vi "Set_Compliance_Slope_R2.vi"(8 "Compliance Slope":u8=128, 9 "DIO Ref Out":T1, 10 "VISA resource name":refnum<visa-resource-name>="ASRL1::INSTR", 11 "Servo ID":string="\u0001") -> (2 "Valid Checksum":bool=TRUE, 3 "Error":u64)   [LabVIEW 2015]
uses:
  <vilib>/myRIO/Instrument Drivers/Onboard IO/DIO/typedefs/DIO Reference.ctl
  <vilib>/myRIO/Common/Instrument Driver Framework/Utilities/typedefs/myRIO Generic Hardware Reference.ctl
  <vilib>/myRIO/Common/Instrument Driver Framework/Utilities/typedefs/Hardware Version Enum.ctl
  <vilib>/myRIO/Common/Instrument Driver Framework/Utilities/typedefs/myRIO v1.0 Reference.ctl
  <vilib>/myRIO/Common/Instrument Driver Framework/Utilities/typedefs/Generic FPGA Reference.ctl
  <vilib>/myRIO/Common/Instrument Driver Framework/myRIO v1.0/DIO/typedefs/DIO Channels List.ctl
  <vilib>/myRIO/Common/Instrument Driver Framework/myRIO v1.0/DIO/typedefs/DIO Channels Enum.ctl
  <vilib>/Utility/error.llb/Error Cluster From Error Code.vi
  <vilib>/myRIO/Common/Instrument Driver Framework/myRIO v1.0/DIO/vis/myRIO v1.0 Write DIO.vi
  <vilib>/myRIO/Instrument Drivers/Onboard IO/DIO/DIO.lvlib
panel:
  out "Valid Checksum 2":bool=TRUE
  out "Error 2":u64
  out "Received String 2":string
  out "Received String Array 2":string[](array[string])
  out "Received\nArray 2":u8[](array[numeric])
  out "Received\nCksm 2":u8
  out "Calc Cksm 2":u8
  in  "Return\nDelay (us) 2":i32=1000
  in  "RECEIVE (F) 2":bool[](array[boolean])=[FALSE]
  out "Tx Packet 2":string
  out "Checksum 2":string
  in  "Transmit \nDelay (us) 2":i32=850
  out "CS 2":string
  in  "TRANSMIT (T) 2":bool[](array[boolean])=[TRUE]
  out "CS":string
  out "Checksum":string
  out "Tx Packet":string
  out "Calc Cksm":u8
  out "Received\nCksm":u8
  out "Received\nArray":u8[](array[numeric])
  in  "Transmit \nDelay (us)":i32=850
  in  "Return\nDelay (us)":i32=1000
  in  "RECEIVE (F)":bool[](array[boolean])=[FALSE]
  in  "TRANSMIT (T)":bool[](array[boolean])=[TRUE]
  out "Received String Array":string[](array[string])
  out "Received String":string
  # "SEND VALUES"
  # "RECEIVED VALUES"
  # "OUTPUT VALUES"
  # "INPUT"
  # "Config Parameters"
  # "Tx/Rx Delays"
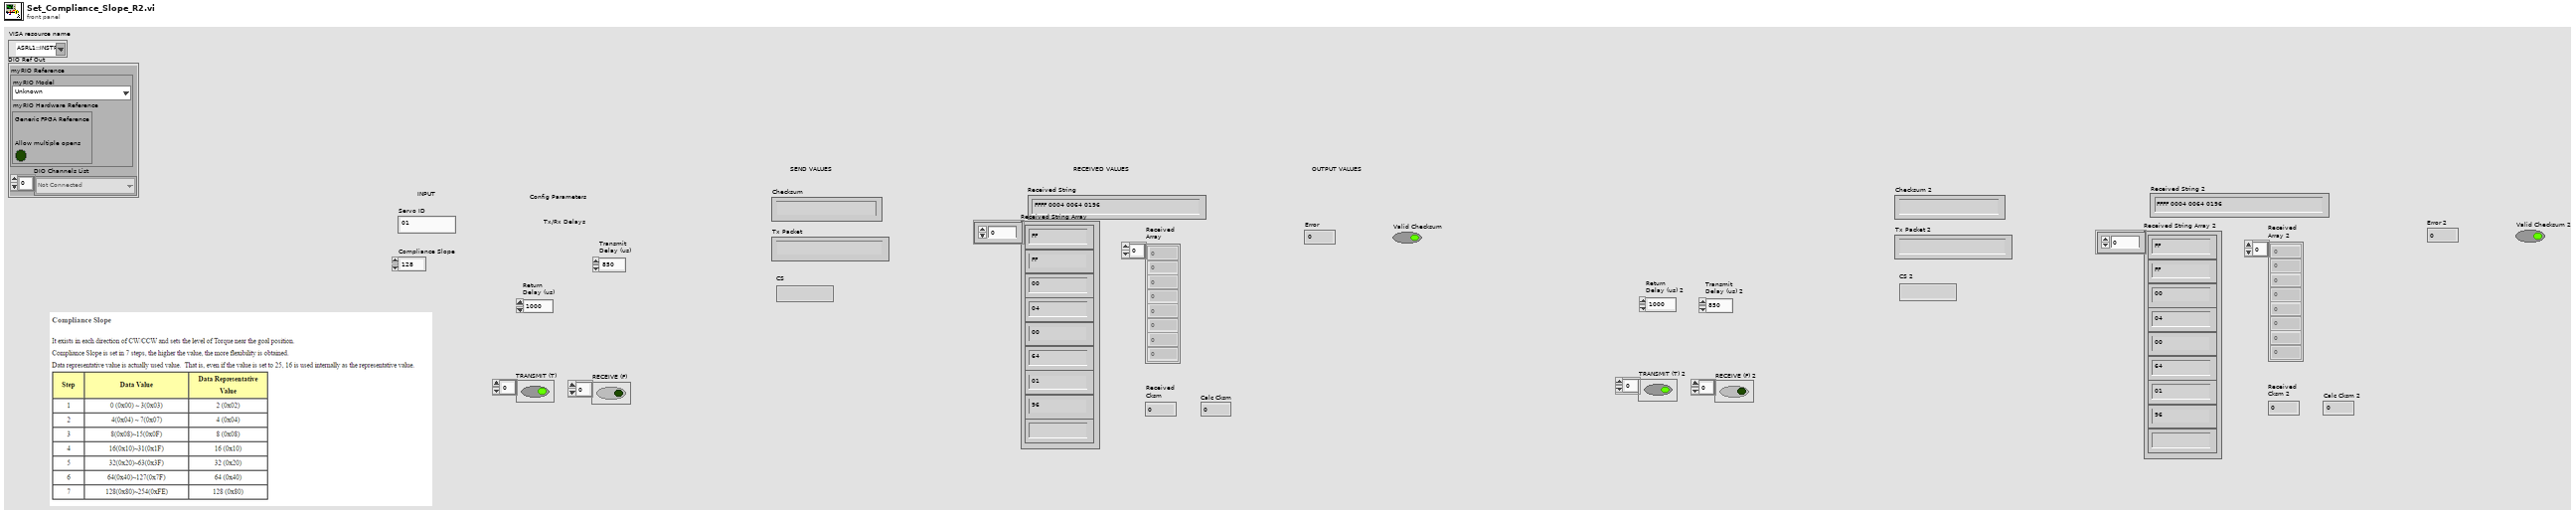
[diagram p1: front panel]
types:
  T1 = typedef "DIO.lvlib/DIO Reference.ctl" = cluster{"myRIO Reference":T2, "DIO Channels List":T6}
  T2 = typedef "myRIO Generic Hardware Reference.ctl" = cluster{"myRIO Model":T3, "myRIO Hardware Reference":T4}
  T3 = typedef "Hardware Version Enum.ctl" = enum16{"Unknown", "myRIO-1900", "myRIO-1950", "roboRIO"}
  T4 = typedef "myRIO v1.0 Reference.ctl" = cluster{"Generic FPGA Reference":T5, "Allow multiple opens":bool}
  T5 = typedef "Generic FPGA Reference.ctl" = refnum<k20>
  T6 = typedef "DIO Channels List.ctl" = T7[]
  T7 = typedef "DIO Channels Enum.ctl" = enum16{"Not Connected", "C/DIO0", "C/DIO1", "C/DIO2", "C/DIO3", "C/DIO4", "C/DIO5", "C/DIO6", "C/DIO7", "A/DIO0", "A/DIO1", "A/DIO2", "A/DIO3", "A/DIO4", "A/DIO5", "A/DIO6", "A/DIO7", "A/DIO8", "A/DIO9", "A/DIO10", "A/DIO11", "A/DIO12", "A/DIO13", "A/DIO14", "A/DIO15", "B/DIO0", "B/DIO1", "B/DIO2", "B/DIO3", "B/DIO4", "B/DIO5", "B/DIO6", "B/DIO7", "B/DIO8", "B/DIO9", "B/DIO10", "B/DIO11", "B/DIO12", "B/DIO13", "B/DIO14", "B/DIO15", "LED0", "LED1", "LED2", "LED3", "Button0", "DIO/DIO0", "DIO/DIO1", "DIO/DIO2", "DIO/DIO3", "DIO/DIO4", "DIO/DIO5", "DIO/DIO6", "DIO/DIO7", "DIO/DIO8", "DIO/DIO9", "SPI/CS0", "SPI/CS1", "SPI/CS2", "SPI/CS3", "LED RADIO (Green)", "LED RADIO (Red)", "LED COMM (Green)", "LED COMM (Red)", "LED MODE (Green)", "LED MODE (Red)"}
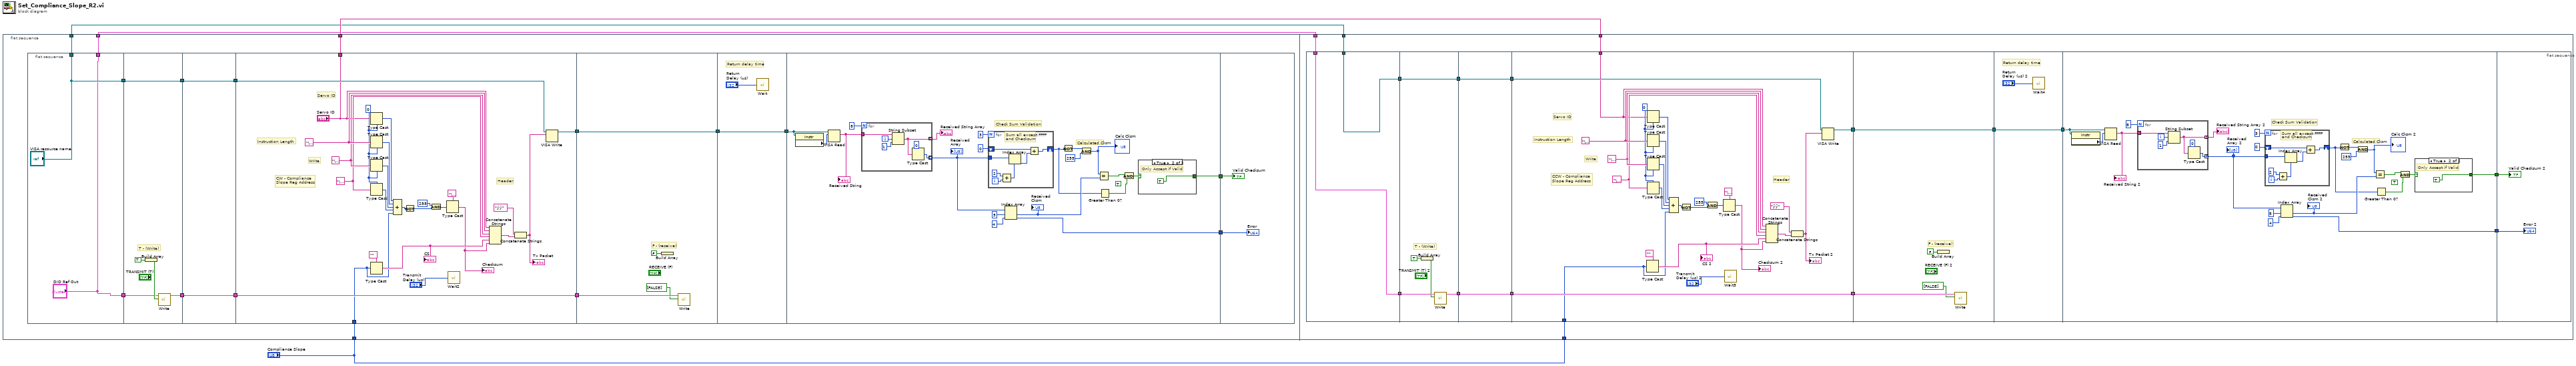
[diagram p0: block diagram]
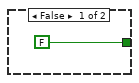
[diagram p2: hidden frame]
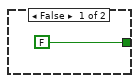
[diagram p3: hidden frame]
diagram:
  n1 = flat-sequence {
    tunnel: "Compliance Slope" -> [w8]
    tunnel: [w7] -> w3
    tunnel: [w5] -> w2
    tunnel: [w6] -> w1
    tunnel: "Compliance Slope" -> [w101]
    tunnel: w3 -> [w100]
    tunnel: w2 -> [w99]
    tunnel: w1 -> [w98]
    frame #0 {
      n2 = flat-sequence {
        tunnel: ["VISA resource name"] -> w20
        tunnel: ["DIO Ref Out"] -> w19
        tunnel: ["DIO Ref Out"] -> w6
        tunnel: ["VISA resource name"] -> w5
        tunnel: [w27] -> w18
        tunnel: [w25] -> w17
        tunnel: w20 -> [w25]
        tunnel: w19 -> [w23]
        tunnel: [w29] -> w16
        tunnel: w18 -> [w29]
        tunnel: [w28] -> w15
        tunnel: w17 -> [w28]
        tunnel: [w54] -> w13
        tunnel: w16 -> [w54]
        tunnel: w15 -> [w53]
        tunnel: [w52] -> w14
        tunnel: w8 -> [w31]
        tunnel: ["Servo ID"] -> w7
        tunnel: [w56] -> w12
        tunnel: w14 -> [w56]
        tunnel: w13 -> [w58]
        tunnel: w12 -> [w59]
        tunnel: [w59] -> w11
        tunnel: w11 -> [w78]
        tunnel: [w63] -> w10
        tunnel: [w61] -> w9
        tunnel: w10 -> [w97]
        tunnel: w9 -> [w96]
        frame #0 {
        }
        frame #1 {
          # "T - (Write)"
          n3 = Build Array(TRUE) -> (w24:bool[])
          n4 = call <vilib>:"Write.vi"("Values"=w24, "DIO Ref In"=w23) -> ("DIO Ref Out"=w27:T1)  [unwired: 7 in, 1 out]
        }
        frame #2 {
        }
        frame #3 {
          w39 = u8 0
          w34 = "\u001c"
          w43 = "\u0003"
          w44 = "\u0004"
          # "CW - Compliance\nSlope Reg Address"
          # "Write"
          # "Instruction Length"
          # "Servo ID"
          # "Header"
          n5 = Type Cast(type="", x=w31) -> (*(type *) &x=w33:string)
          "CS" <- w33
          n6 = Type Cast(type=w39, x="Servo ID") -> (*(type *) &x=w45:u8)
          n7 = Type Cast(type=w39, x=w44) -> (*(type *) &x=w46:u8)
          n8 = Type Cast(type=w39, x=w43) -> (*(type *) &x=w38:u8)
          n9 = Type Cast(type=w39, x=w34) -> (*(type *) &x=w47:u8)
          n10 = Compound Arithmetic op=ADD(w45, w46, w38, w47, w31) -> (w48:u8)
          n11 = Not(x=w48) -> (.not. x?=w50:u8)
          n12 = And(x=u8 255, y=w50) -> (x .and. y?=w51:u8)
          n13 = Type Cast(type="\u0000", x=w51) -> (*(type *) &x=w32:string)
          "Checksum" <- w32
          n14 = call "Wait2"("Count(uSec)"="Transmit \nDelay (us)") -> ()  [unwired: 1 out]
          n15 = Concatenate Strings("Servo ID", w44, w43, w34, w33, w32) -> (w41:string)
          n16 = Concatenate Strings("ÿÿ", w41) -> (w37:string)
          "Tx Packet" <- w37
          n17 = VISA Write(VISA resource name=w53, write buffer=w37) -> (VISA resource name out=w52:refnum<visa-resource-name>)  [unwired: 1 in, 2 out]
        }
        frame #4 {
          # "F - (receive)"
          n18 = Build Array(FALSE) -> ()  [unwired: 1 out]
          n19 = call <vilib>:"Write.vi"("Values"=bool[] [FALSE], "DIO Ref In"=w58) -> ()  [unwired: 7 in, 2 out]
        }
        frame #5 {
          # "Return delay time"
          n20 = call "Wait"("Count(uSec)"="Return\nDelay (us)") -> ()  [unwired: 1 out]
        }
        frame #6 {
          (unwired) TRUE
          # "Calculated Cksm"
          # "Check Sum Validation"
          n21 = property class="Instr"(reference=w78) -> ("Serial Settings:Number of Bytes at Serial Port"=w77:u32)  [unwired: 1 in, 2 out]
          n22 = VISA Read(VISA resource name=w78, byte count=w77) -> (read buffer=w79:string)  [unwired: 1 in, 3 out]
          "Received String" <- w79
          n23 = for {
            N: 8 -> [_]
            tunnel: w79 -> [w95]
            tunnel: [w91] -> w76 mode=indexing
            tunnel: [w90] -> w74 mode=indexing
            i -> [w94]
            n24 = String Subset(string=w95, offset (0)=w94, length (rest)=1) -> (substring=w91:string)
            n25 = Type Cast(type=u8 0, x=w91) -> (*(type *) &x=w90:u8)
          }
          "Received String Array" <- w76
          "Received\nArray" <- w74
          n26 = for {
            N: 3 -> [_]
            tunnel: w74 -> [w86]
            shift-right: [w85] -> w67
            shift-left: u8 0 -> [w84]
            i -> [w89]
            # "Sum all except FFFF\nand Checksum"
            n27 = Add(x=2, y=w89) -> (x+y=w87:i32)
            n28 = Index Array(array=w86, index=w87) -> (element=w83:u8)
            n29 = Add(x=w84, y=w83) -> (x+y=w85:u8)
          }
          n30 = Index Array(array=w74, index #1=5 ("x"), index #2=4 ("x")) -> (element #1=w68:u8, element #2=w61:u8)
          "Received\nCksm" <- w68
          n31 = Not(x=w67) -> (.not. x?=w71:u8)
          n32 = And(x=w71, y=u8 255) -> (x .and. y?=w69:u8)
          "Calc Cksm" <- w69
          n33 = Equal?(x=w69, y=w68) -> (x = y?=w65:bool)
          n34 = Greater Than 0?(x=w67) -> (x > 0?=w64:bool)
          n35 = And(x=w65, y=w64) -> (x .and. y?=w66:bool)
          n36 = case shown="True" w66 {
            tunnel: [FALSE TRUE] -> w63
            frame False {
            }
            frame True {
              # "Only Accept if Valid"
            }
          }
        }
        frame #7 {
          "Valid Checksum" <- w97
          "Error" <- w96
        }
      }
    }
    frame #1 {
      n37 = flat-sequence {
        tunnel: [w115] -> w113
        tunnel: [w114] -> w112
        tunnel: w99 -> [w115]
        tunnel: w98 -> [w114]
        tunnel: [w120] -> w111
        tunnel: [w118] -> w110
        tunnel: w113 -> [w118]
        tunnel: w112 -> [w116]
        tunnel: [w122] -> w109
        tunnel: w111 -> [w122]
        tunnel: [w121] -> w108
        tunnel: w110 -> [w121]
        tunnel: [w147] -> w106
        tunnel: w109 -> [w147]
        tunnel: w108 -> [w146]
        tunnel: [w145] -> w107
        tunnel: w101 -> [w124]
        tunnel: w100 -> [w123]
        tunnel: [w149] -> w105
        tunnel: w107 -> [w149]
        tunnel: w106 -> [w151]
        tunnel: w105 -> [w152]
        tunnel: [w152] -> w104
        tunnel: w104 -> [w171]
        tunnel: [w156] -> w103
        tunnel: [w154] -> w102
        tunnel: w103 -> [w190]
        tunnel: w102 -> [w189]
        frame #0 {
        }
        frame #1 {
          # "T - (Write)"
          n38 = Build Array(TRUE) -> (w117:bool[])
          n39 = call <vilib>:"Write.vi"("Values"=w117, "DIO Ref In"=w116) -> ("DIO Ref Out"=w120:T1)  [unwired: 7 in, 1 out]
        }
        frame #2 {
        }
        frame #3 {
          w132 = u8 0
          w127 = "\u001d"
          w136 = "\u0003"
          w137 = "\u0004"
          # "CCW - Compliance\nSlope Reg Address"
          # "Write"
          # "Instruction Length"
          # "Servo ID"
          # "Header"
          n40 = Type Cast(type="", x=w124) -> (*(type *) &x=w126:string)
          "CS 2" <- w126
          n41 = Type Cast(type=w132, x=w123) -> (*(type *) &x=w138:u8)
          n42 = Type Cast(type=w132, x=w137) -> (*(type *) &x=w139:u8)
          n43 = Type Cast(type=w132, x=w136) -> (*(type *) &x=w131:u8)
          n44 = Type Cast(type=w132, x=w127) -> (*(type *) &x=w140:u8)
          n45 = Compound Arithmetic op=ADD(w138, w139, w131, w140, w124) -> (w141:u8)
          n46 = Not(x=w141) -> (.not. x?=w143:u8)
          n47 = And(x=u8 255, y=w143) -> (x .and. y?=w144:u8)
          n48 = Type Cast(type="\u0000", x=w144) -> (*(type *) &x=w125:string)
          "Checksum 2" <- w125
          n49 = call "Wait3"("Count(uSec)"="Transmit \nDelay (us) 2") -> ()  [unwired: 1 out]
          n50 = Concatenate Strings(w123, w137, w136, w127, w126, w125) -> (w134:string)
          n51 = Concatenate Strings("ÿÿ", w134) -> (w130:string)
          "Tx Packet 2" <- w130
          n52 = VISA Write(VISA resource name=w146, write buffer=w130) -> (VISA resource name out=w145:refnum<visa-resource-name>)  [unwired: 1 in, 2 out]
        }
        frame #4 {
          # "F - (receive)"
          n53 = Build Array(FALSE) -> ()  [unwired: 1 out]
          n54 = call <vilib>:"Write.vi"("Values"=bool[] [FALSE], "DIO Ref In"=w151) -> ()  [unwired: 7 in, 2 out]
        }
        frame #5 {
          # "Return delay time"
          n55 = call "Wait4"("Count(uSec)"="Return\nDelay (us) 2") -> ()  [unwired: 1 out]
        }
        frame #6 {
          (unwired) TRUE
          # "Calculated Cksm"
          # "Check Sum Validation"
          n56 = property class="Instr"(reference=w171) -> ("Serial Settings:Number of Bytes at Serial Port"=w170:u32)  [unwired: 1 in, 2 out]
          n57 = VISA Read(VISA resource name=w171, byte count=w170) -> (read buffer=w172:string)  [unwired: 1 in, 3 out]
          "Received String 2" <- w172
          n58 = for {
            N: 8 -> [_]
            tunnel: w172 -> [w188]
            tunnel: [w184] -> w169 mode=indexing
            tunnel: [w183] -> w167 mode=indexing
            i -> [w187]
            n59 = String Subset(string=w188, offset (0)=w187, length (rest)=1) -> (substring=w184:string)
            n60 = Type Cast(type=u8 0, x=w184) -> (*(type *) &x=w183:u8)
          }
          "Received String Array 2" <- w169
          "Received\nArray 2" <- w167
          n61 = for {
            N: 3 -> [_]
            tunnel: w167 -> [w179]
            shift-right: [w178] -> w160
            shift-left: u8 0 -> [w177]
            i -> [w182]
            # "Sum all except FFFF\nand Checksum"
            n62 = Add(x=2, y=w182) -> (x+y=w180:i32)
            n63 = Index Array(array=w179, index=w180) -> (element=w176:u8)
            n64 = Add(x=w177, y=w176) -> (x+y=w178:u8)
          }
          n65 = Index Array(array=w167, index #1=5 ("x"), index #2=4 ("x")) -> (element #1=w161:u8, element #2=w154:u8)
          "Received\nCksm 2" <- w161
          n66 = Not(x=w160) -> (.not. x?=w164:u8)
          n67 = And(x=w164, y=u8 255) -> (x .and. y?=w162:u8)
          "Calc Cksm 2" <- w162
          n68 = Equal?(x=w162, y=w161) -> (x = y?=w158:bool)
          n69 = Greater Than 0?(x=w160) -> (x > 0?=w157:bool)
          n70 = And(x=w158, y=w157) -> (x .and. y?=w159:bool)
          n71 = case shown="True" w159 {
            tunnel: [FALSE TRUE] -> w156
            frame False {
            }
            frame True {
              # "Only Accept if Valid"
            }
          }
        }
        frame #7 {
          "Valid Checksum 2" <- w190
          "Error 2" <- w189
        }
      }
    }
  }
